vi "function_timer_stop.vi"(10 "s<=2?":bool, 11 "x":dbl) -> (3 "Count":dbl)   [LabVIEW 2018]
panel:
  out "Second":dbl
  in  "stop":bool
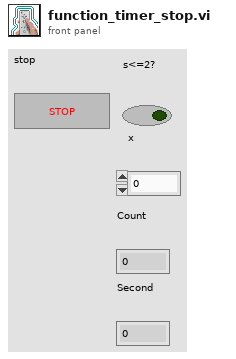
[diagram p1: front panel]
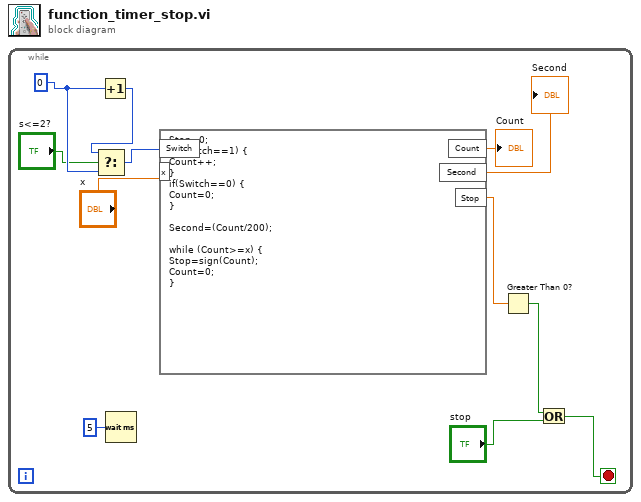
[diagram p0: block diagram]
diagram:
  n1 = while {
    stop <- w4 stop-if-true
    w9 = 0
    n2 = Increment(x=w9) -> (x+1=w10:i32)
    n3 = Select(t=w10, s="s<=2?", f=w9) -> (s? t:f=w11:i32)
    n4 = Wait (ms)(milliseconds to wait=u32 5) -> ()  [unwired: 1 out]
    n5 = formula code="Stop=0;\nif (Switch==1) {\nCount++;\n}\nif(Switch==0) {\nCount=0;\n}\n\nSecond=(Count/200);\n\nwhile (Count>=x) {\nStop=sign(Count);\nCount=0;\n}"("Switch"=w11, "x"="x") -> ("Count"=→"Count":dbl, "Second"=→"Second":dbl, "Stop"=w6:dbl)
    n6 = Greater Than 0?(x=w6) -> (x > 0?=w5:bool)
    n7 = Or(x=w5, y="stop") -> (x .or. y?=w4:bool)
  }
